vi "Describe VI Refnum Failure.vi"(1 "Expected":refnum<vi>, 2 "Got":refnum<vi>) -> (0 "Failure Description":string)   [LabVIEW 2013]
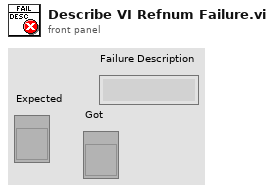
[diagram p1: front panel]
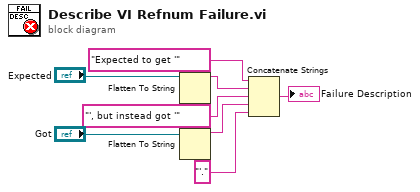
[diagram p0: block diagram]
diagram:
  n1 = Flatten To String(anything="Expected") -> (data string=w4:string)  [unwired: 3 in, 2 out]
  n2 = Flatten To String(anything="Got") -> (data string=w3:string)  [unwired: 3 in, 2 out]
  n3 = Concatenate Strings("Expected to get '", w4, "', but instead got '", w3, "'.") -> (→"Failure Description":string)
